vi "Parse CfgTable(with DataName).vi"(5 "Format":string, 6 "Array delimiters (|)":string="|", 7 "Cluster Configuration Typedef":variant, 8 "error in (no error)":errorcluster, 11 "CfgTable Row":string[](array[string])) -> (0 "error out":errorcluster, 1 "Elements":i32, 3 "Cluster Configuration Out":variant)   [LabVIEW 2017, in "ClusterCfgTable.lvlib"]
doc: "Parses a configuration table back into a cluster, using the data names recorded in the table to place each value. The cluster type comes from Cluster Configuration Typedef, and Elements reports how many elements were read."
uses:
  ClusterCfgTable.lvlib
  <vilib>/Utility/Data Type/Type Definitions/Data Type.ctl
  <vilib>/Utility/Data Type/Type Definitions/Refnum Type.ctl
  <vilib>/Utility/Data Type/NI_Data Type.lvlib
  _openG/_reuse_openG.lvlib
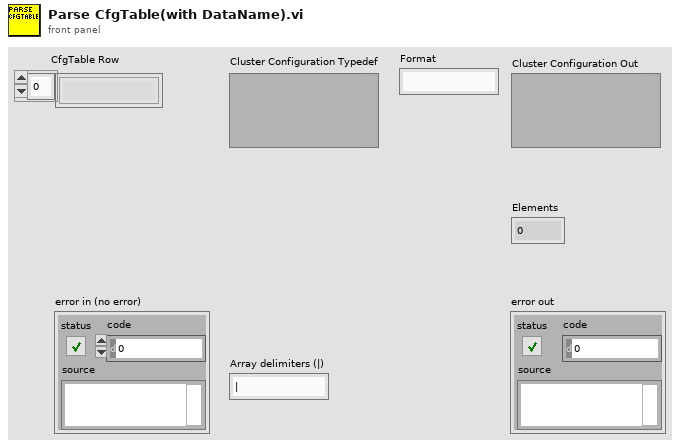
[diagram p1: front panel]
types:
  T1 = typedef "NI_Data Type.lvlib/Data Type.ctl" = enum8{"Invalid Type", "Void", "I8", "I16", "I32", "I64", "U8", "U16", "U32", "U64", "Single Float", "Double Float", "Extended Float", "Single Complex", "Double Complex", "Extended Complex", "Enum U8", "Enum U16", "Enum U32", "Enum U64", "Single Float With Unit", "Double Float With Unit", "Extended Float With Unit", "Single Complex with Unit", "Double Complex with Unit", "Extended Complex with Unit", "Boolean", "String", "Path", "Picture", "Tag", "Array", "Cluster", "Variant", "LV Variant", "Waveform", "Timestamp", "Digital Waveform", "Digital Data", "ExpressData", "Refnum", "External Data", "VI", "Poly VI", "LabVIEW Class Instance", "Fixed Point"}
  T2 = typedef "NI_Data Type.lvlib/Refnum Type.ctl" = enum16{"NotARefnum", "UnknownRefnum", "Generic", "Datalog", "ByteStream", "Device", "Occurence", "TCPNetConnection", "Auto", "Menu", "Imaq", "Hardware", "DataSocket", "Visa", "IVI", "UDPNetConnection", "Notifier", "Queue", "Irda", "EventReg", "DotNet", "UserEvent", "Callback", "UNUSED_EMPTY_POSITION", "BlueToothNetConnection", "LVObjApp", "LVObjVI", "LVObjUnknown", "GenericClass", "UserDefinedRefnumTag", "DataValue", "RT FIFO", "TDMS File"}
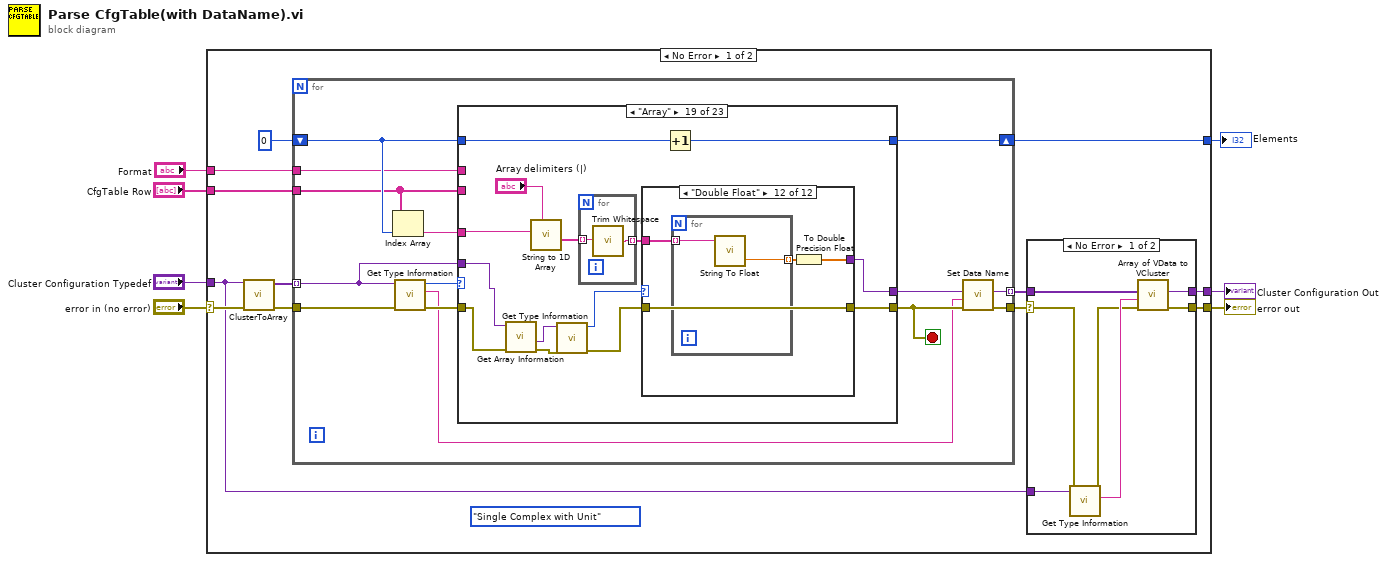
[diagram p0: block diagram]
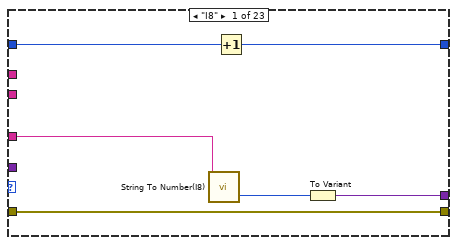
[diagram p3: hidden frame]
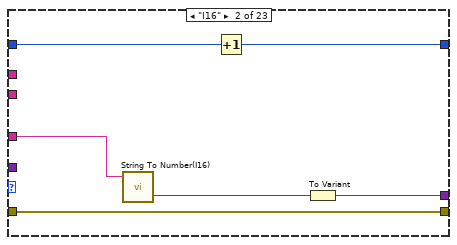
[diagram p4: hidden frame]
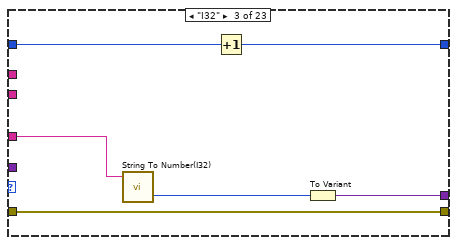
[diagram p5: hidden frame]
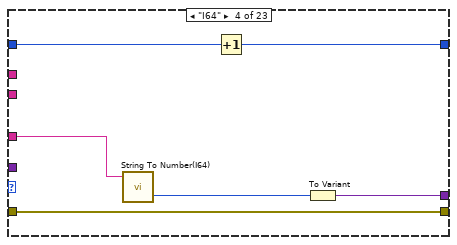
[diagram p6: hidden frame]
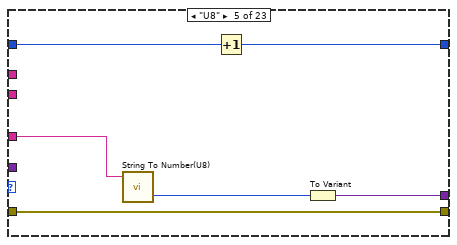
[diagram p7: hidden frame]
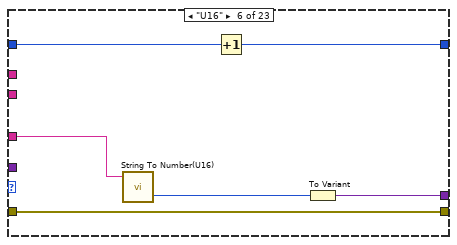
[diagram p8: hidden frame]
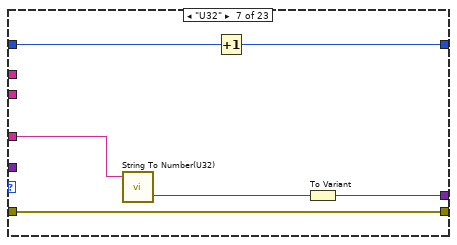
[diagram p9: hidden frame]
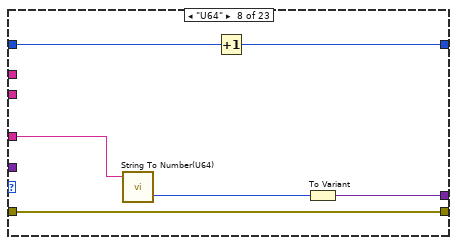
[diagram p10: hidden frame]
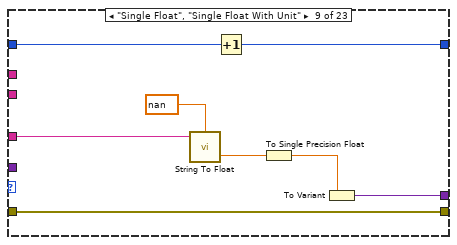
[diagram p11: hidden frame]
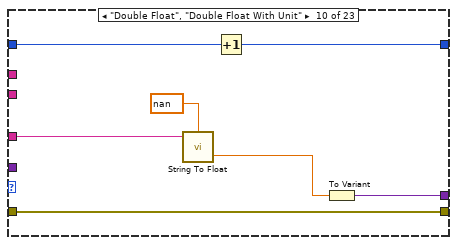
[diagram p12: hidden frame]
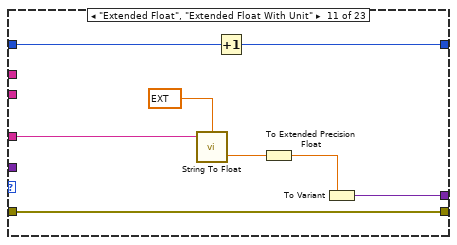
[diagram p13: hidden frame]
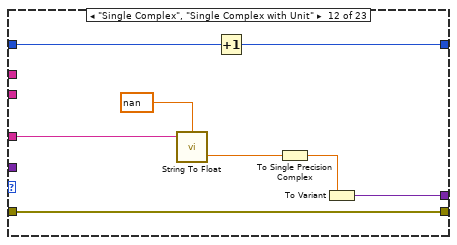
[diagram p14: hidden frame]
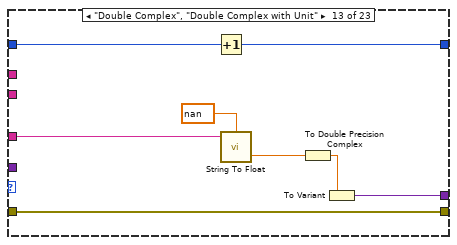
[diagram p15: hidden frame]
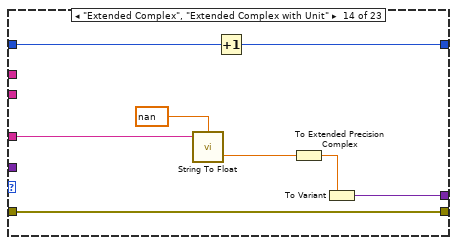
[diagram p16: hidden frame]
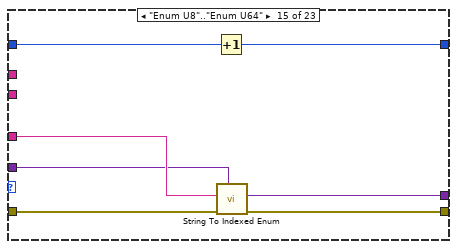
[diagram p17: hidden frame]
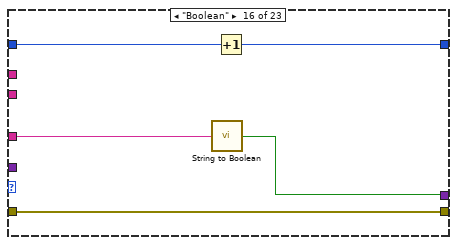
[diagram p18: hidden frame]
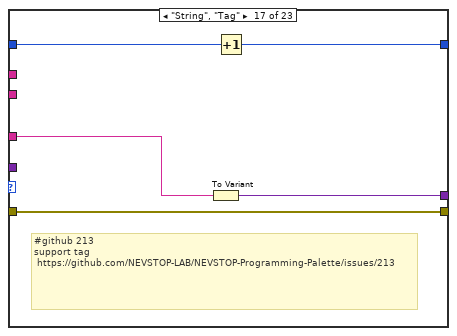
[diagram p19: hidden frame]
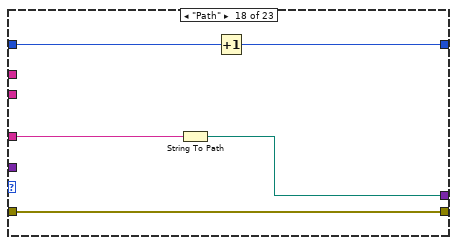
[diagram p20: hidden frame]
diagram:
  n1 = case shown="No Error" "error in (no error)" {
    selector: "error in (no error)" -> [w14 w284]
    tunnel: "CfgTable Row" -> [w19 _]
    tunnel: [w18 w283] -> w6
    tunnel: [w17 w284] -> w5
    tunnel: "Cluster Configuration Typedef" -> [w10 w283]
    tunnel: [w9 _] -> w2
    tunnel: "Format" -> [w8 _]
    frame No Error {
      (unwired) Data_Type."Single Complex with Unit" ("Type")
      n2 = call "ClusterToArray.vi"("Error in"=w14, "Cluster"=w10) -> ("Error out"=w15:errorcluster, "Array"=w12:variant[])  [unwired: 8 in]
      n3 = for {
        tunnel: w19 -> [w38]
        tunnel: w12 -> [w34] mode=indexing
        tunnel: [w37] -> w13 mode=indexing
        tunnel: w15 -> [w32]
        tunnel: [w35] -> w16
        shift-right: [w40] -> w9
        shift-left: 0 -> [w39]
        tunnel: w8 -> [w30]
        stop <- w36 stop-if-true
        n4 = Index Array(array=w38, index=w39) -> (element=w42:string)
        n5 = call <vilib>:"Get Type Information.vi"("error in (no error)"=w32, "Variant"=w34) -> ("error out"=w31:errorcluster, "Name"=w29:string, "Type"=w33:T1)  [unwired: 5 in, 2 out]
        n6 = case shown="\"Array\"" w33 {
          tunnel: w42 -> [w43 w49 w55 w61 w67 w73 w79 w85 w97 w100 w112 w120 w128 w136 w144 w149 w154 w157 w171 _ w250 w260 _]
          tunnel: [w48 w54 w60 w66 w72 w78 w84 w90 w98 w105 w113 w121 w129 w137 w143 w148 w153 w156 w168 w239 w251 w261 w277] -> w41
          tunnel: w34 -> [_ _ _ _ _ _ _ _ _ _ _ _ _ _ w142 _ _ _ w162 w240 _ w262 w277]
          tunnel: w31 -> [w46 w52 w58 w64 w70 w76 w82 w88 w96 w104 w111 w119 w127 w135 w141 w147 w152 w155 w163 w243 w245 w267 w282]
          tunnel: [w46 w52 w58 w64 w70 w76 w82 w88 w96 w104 w111 w119 w127 w135 w140 w147 w152 w155 w166 w236 w244 w266 w281] -> w36
          tunnel: w39 -> [w45 w51 w57 w63 w69 w75 w81 w87 w95 w103 w110 w118 w126 w134 w139 w146 w151 w159 w173 w238 w249 w265 w276]
          tunnel: [w44 w50 w56 w62 w68 w74 w80 w86 w94 w102 w109 w117 w125 w133 w138 w145 w150 w158 w172 w237 w248 w265 w276] -> w40
          tunnel: w38 -> [_ _ _ _ _ _ _ _ _ _ _ _ _ _ _ _ _ _ _ w242 _ _ _]
          tunnel: w30 -> [_ _ _ _ _ _ _ _ _ _ _ _ _ _ _ _ _ _ _ _ w246 _ _]
          frame "I8" {
            n7 = call "String To Number(I8).vi"("String"=w43) -> ("Numeric(I8)"=w47:i8)  [unwired: 4 in]
            n8 = Increment(x=w45) -> (x+1=w44:i32)
            n9 = To Variant(anything=w47) -> (Variant=w48:variant)
          }
          frame "I16" {
            n10 = call "String To Number(I16).vi"("String"=w49) -> ("Numeric(I16)"=w53:i16)  [unwired: 4 in]
            n11 = Increment(x=w51) -> (x+1=w50:i32)
            n12 = To Variant(anything=w53) -> (Variant=w54:variant)
          }
          frame "I32" {
            n13 = call "String To Number(I32).vi"("String"=w55) -> ("Numeric(I32)"=w59:i32)  [unwired: 4 in]
            n14 = Increment(x=w57) -> (x+1=w56:i32)
            n15 = To Variant(anything=w59) -> (Variant=w60:variant)
          }
          frame "I64" {
            n16 = call "String To Number(I64).vi"("String"=w61) -> ("Numeric(I64)"=w65:i64)  [unwired: 4 in]
            n17 = Increment(x=w63) -> (x+1=w62:i32)
            n18 = To Variant(anything=w65) -> (Variant=w66:variant)
          }
          frame "U8" {
            n19 = call "String To Number(U8).vi"("String"=w67) -> ("Numeric(U8)"=w71:u8)  [unwired: 4 in]
            n20 = Increment(x=w69) -> (x+1=w68:i32)
            n21 = To Variant(anything=w71) -> (Variant=w72:variant)
          }
          frame "U16" {
            n22 = call "String To Number(U16).vi"("String"=w73) -> ("Numeric(U16)"=w77:u16)  [unwired: 4 in]
            n23 = Increment(x=w75) -> (x+1=w74:i32)
            n24 = To Variant(anything=w77) -> (Variant=w78:variant)
          }
          frame "U32" {
            n25 = call "String To Number(U32).vi"("String"=w79) -> ("Numeric(U32)"=w83:u32)  [unwired: 4 in]
            n26 = Increment(x=w81) -> (x+1=w80:i32)
            n27 = To Variant(anything=w83) -> (Variant=w84:variant)
          }
          frame "U64" {
            n28 = call "String To Number(U64).vi"("String"=w85) -> ("Numeric(U64)"=w89:u64)  [unwired: 4 in]
            n29 = Increment(x=w87) -> (x+1=w86:i32)
            n30 = To Variant(anything=w89) -> (Variant=w90:variant)
          }
          frame "Single Float", "Single Float With Unit" {
            n31 = call "String To Float.vi"("Default(0)"=nan ("number"), "String"=w97) -> ("Float"=w93:dbl)  [unwired: 3 in]
            n32 = Increment(x=w95) -> (x+1=w94:i32)
            n33 = To Single Precision Float(number=w93) -> (single precision float=w92:sgl)
            n34 = To Variant(anything=w92) -> (Variant=w98:variant)
          }
          frame "Double Float", "Double Float With Unit" {
            n35 = call "String To Float.vi"("Default(0)"=nan ("number"), "String"=w100) -> ("Float"=w99:dbl)  [unwired: 3 in]
            n36 = Increment(x=w103) -> (x+1=w102:i32)
            n37 = To Variant(anything=w99) -> (Variant=w105:variant)
          }
          frame "Extended Float", "Extended Float With Unit" {
            n38 = call "String To Float.vi"("Default(0)"=ext nan ("number"), "String"=w112) -> ("Float"=w108:dbl)  [unwired: 3 in]
            n39 = Increment(x=w110) -> (x+1=w109:i32)
            n40 = To Extended Precision Float(1:w108) -> (0:w107:ext)
            n41 = To Variant(anything=w107) -> (Variant=w113:variant)
          }
          frame "Single Complex", "Single Complex with Unit" {
            n42 = call "String To Float.vi"("Default(0)"=nan ("number"), "String"=w120) -> ("Float"=w116:dbl)  [unwired: 3 in]
            n43 = Increment(x=w118) -> (x+1=w117:i32)
            n44 = To Single Precision Complex(1:w116) -> (0:w115:csg)
            n45 = To Variant(anything=w115) -> (Variant=w121:variant)
          }
          frame "Double Complex", "Double Complex with Unit" {
            n46 = Increment(x=w126) -> (x+1=w125:i32)
            n47 = call "String To Float.vi"("Default(0)"=nan ("number"), "String"=w128) -> ("Float"=w124:dbl)  [unwired: 3 in]
            n48 = To Double Precision Complex(1:w124) -> (0:w123:cdb)
            n49 = To Variant(anything=w123) -> (Variant=w129:variant)
          }
          frame "Extended Complex", "Extended Complex with Unit" {
            n50 = call "String To Float.vi"("Default(0)"=nan ("number"), "String"=w136) -> ("Float"=w132:dbl)  [unwired: 3 in]
            n51 = Increment(x=w134) -> (x+1=w133:i32)
            n52 = To Extended Precision Complex(1:w132) -> (0:w131:cxt)
            n53 = To Variant(anything=w131) -> (Variant=w137:variant)
          }
          frame "Enum U8".."Enum U64" {
            n54 = Increment(x=w139) -> (x+1=w138:i32)
            n55 = call "String To Indexed Enum.vi"("Variant"=w142, "error in (no error)"=w141, "String"=w144) -> ("error out"=w140:errorcluster, "Enum"=w143:variant)  [unwired: 7 in]
          }
          frame "Boolean" {
            n56 = call "String to Boolean.vi"("String"=w149) -> ("Boolean"=w148:bool)  [unwired: 3 in]
            n57 = Increment(x=w146) -> (x+1=w145:i32)
          }
          frame "String", "Tag" {
            # "#github 213\nsupport tag\n https://github.com/NEVSTOP-LAB/NEVSTOP-Programming-Palette/issues/213"
            n58 = To Variant(anything=w154) -> (Variant=w153:variant)
            n59 = Increment(x=w151) -> (x+1=w150:i32)
          }
          frame "Path" {
            n60 = String To Path(string=w157) -> (path=w156:path)
            n61 = Increment(x=w159) -> (x+1=w158:i32)
          }
          frame "Array" {
            n62 = call <vilib>:"Get Array Information.vi"("error in (no error)"=w163, "Variant"=w162) -> ("error out"=w165:errorcluster, "Array Element Data Type"=w164:variant)  [unwired: 6 in, 2 out]
            n63 = call "String to 1D Array.vi"("delimiter (Tab)"="Array delimiters (|)", "string"=w171) -> ("Array of Strings"=w169:string[])  [unwired: 9 in]
            n64 = call <vilib>:"Get Type Information.vi"("error in (no error)"=w165, "Variant"=w164) -> ("error out"=w161:errorcluster, "Type"=w160:T1)  [unwired: 5 in, 3 out]
            n65 = for {
              tunnel: w169 -> [w175] mode=indexing
              tunnel: [w174] -> w167 mode=indexing
              n66 = call <vilib>:"Trim Whitespace.vi"("string"=w175) -> ("trimmed string"=w174:string)  [unwired: 1 in]
            }
            n67 = case shown="\"Double Float\"" w160 {
              tunnel: [w179 w180 w183 w188 w193 w198 w203 w208 w213 w218 w223 w229] -> w168
              tunnel: w167 -> [w179 w182 w185 w190 w195 w200 w205 w210 w215 w220 w226 w232]
              tunnel: [w176 w181 w184 w189 w194 w199 w204 w209 w214 w219 w225 w231] -> w166
              tunnel: w161 -> [_ w181 w184 w189 w194 w199 w204 w209 w214 w219 w225 w231]
              frame "Invalid Type", Default {
                n68 = call "Error From Error Code.vi"("error message (\"\")"="Input Config Contains unsupported datatype" ("String to Prepend to source (\"\")"), "error code (0)"=1 ("code")) -> ("error out"=w176:errorcluster)  [unwired: 7 in]
              }
              frame "String" {
                n69 = To Variant(anything=w182) -> (Variant=w180:variant)
              }
              frame "U8" {
                n70 = for {
                  tunnel: w185 -> [w187] mode=indexing
                  tunnel: [w186] -> w183 mode=indexing
                  n71 = call "String To Number(U8).vi"("String"=w187) -> ("Numeric(U8)"=w186:u8)  [unwired: 4 in]
                }
              }
              frame "U16" {
                n72 = for {
                  tunnel: w190 -> [w192] mode=indexing
                  tunnel: [w191] -> w188 mode=indexing
                  n73 = call "String To Number(U16).vi"("String"=w192) -> ("Numeric(U16)"=w191:u16)  [unwired: 4 in]
                }
              }
              frame "U32" {
                n74 = for {
                  tunnel: w195 -> [w197] mode=indexing
                  tunnel: [w196] -> w193 mode=indexing
                  n75 = call "String To Number(U32).vi"("String"=w197) -> ("Numeric(U32)"=w196:u32)  [unwired: 4 in]
                }
              }
              frame "U64" {
                n76 = for {
                  tunnel: w200 -> [w202] mode=indexing
                  tunnel: [w201] -> w198 mode=indexing
                  n77 = call "String To Number(U64).vi"("String"=w202) -> ("Numeric(U64)"=w201:u64)  [unwired: 4 in]
                }
              }
              frame "I8" {
                n78 = for {
                  tunnel: w205 -> [w207] mode=indexing
                  tunnel: [w206] -> w203 mode=indexing
                  n79 = call "String To Number(I8).vi"("String"=w207) -> ("Numeric(I8)"=w206:i8)  [unwired: 4 in]
                }
              }
              frame "I16" {
                n80 = for {
                  tunnel: w210 -> [w212] mode=indexing
                  tunnel: [w211] -> w208 mode=indexing
                  n81 = call "String To Number(I16).vi"("String"=w212) -> ("Numeric(I16)"=w211:i16)  [unwired: 4 in]
                }
              }
              frame "I32" {
                n82 = for {
                  tunnel: w215 -> [w217] mode=indexing
                  tunnel: [w216] -> w213 mode=indexing
                  n83 = call "String To Number(I32).vi"("String"=w217) -> ("Numeric(I32)"=w216:i32)  [unwired: 4 in]
                }
              }
              frame "I64" {
                n84 = for {
                  tunnel: w220 -> [w222] mode=indexing
                  tunnel: [w221] -> w218 mode=indexing
                  n85 = call "String To Number(I64).vi"("String"=w222) -> ("Numeric(I64)"=w221:i64)  [unwired: 4 in]
                }
              }
              frame "Single Float" {
                n86 = for {
                  tunnel: w226 -> [w228] mode=indexing
                  tunnel: [w227] -> w224 mode=indexing
                  n87 = call "String To Float.vi"("String"=w228) -> ("Float"=w227:dbl)  [unwired: 4 in]
                }
                n88 = To Single Precision Float(number=w224) -> (single precision float=w223:sgl[])
              }
              frame "Double Float" {
                n89 = for {
                  tunnel: w232 -> [w234] mode=indexing
                  tunnel: [w233] -> w230 mode=indexing
                  n90 = call "String To Float.vi"("String"=w234) -> ("Float"=w233:dbl)  [unwired: 4 in]
                }
                n91 = To Double Precision Float(number=w230) -> (double precision float=w229:dbl[])
              }
            }
            n92 = Increment(x=w173) -> (x+1=w172:i32)
          }
          frame "Cluster" {
            n93 = Array Subset(array=w242, index=w238) -> (w241:string[])  [unwired: 1 in]
            n94 = call "Parse CfgTable(with DataName).vi"("Cluster Configuration Typedef"=w240, "error in (no error)"=w243, "CfgTable Row"=w241) -> ("error out"=w236:errorcluster, "Elements"=w235:i32, "Cluster Configuration Out"=w239:variant)  [unwired: 6 in]
            n95 = Add(x=w238, y=w235) -> (x+y=w237:i32)
          }
          frame "Timestamp" {
            n96 = case shown="Default" w250 {
              selector: w250 -> [_ w259]
              tunnel: [timestamp(0 s since 1904-01-01) ("Time Stamp") w257] -> w247
              tunnel: w246 -> [_ w258]
              tunnel: w245 -> [w252 w255]
              tunnel: [w252 w254] -> w244
              frame "" {
              }
              frame Default {
                n97 = Scan From String(format string=w258, input string=w259, error in=w255, default 1=timestamp(0 s since 1904-01-01) ("Time Stamp")) -> (error out=w254:errorcluster, output 1=w257:timestamp)  [unwired: 1 in, 2 out]
              }
            }
            n98 = Increment(x=w249) -> (x+1=w248:i32)
            n99 = To Variant(anything=w247) -> (Variant=w251:variant)
          }
          frame "Refnum" {
            n100 = call <vilib>:"Get Refnum Information.vi"("error in (no error)"=w267, "Variant"=w262) -> ("error out"=w264:errorcluster, "Reference Type"=w263:T2)  [unwired: 6 in, 2 out]
            n101 = case shown="Default" w263 {
              tunnel: [w269 w275] -> w266
              tunnel: w264 -> [w269 w271]
              tunnel: w262 -> [_ w270]
              tunnel: [w268 w270] -> w261
              tunnel: w260 -> [w268 _]
              frame "UserDefinedRefnumTag" {
                (unwired) Refnum_Type."NotARefnum" ("Reference Type")
              }
              frame Default {
                n102 = call "Error From Error Code.vi"("error message (\"\")"="Input Config Contains unsupported datatype" ("String to Prepend to source (\"\")"), "error code (0)"=1 ("code")) -> ("error out"=w274:errorcluster)  [unwired: 7 in]
                n103 = Merge Errors(w271, w274) -> (w275:errorcluster)
              }
            }
          }
          frame Default {
            n104 = call "Error From Error Code.vi"("error message (\"\")"="Input Config Contains unsupported datatype" ("String to Prepend to source (\"\")"), "error code (0)"=1 ("code")) -> ("error out"=w280:errorcluster)  [unwired: 7 in]
            n105 = Merge Errors(w282, w280) -> (w281:errorcluster)
          }
        }
        n106 = call "Set Data Name.vi"("error in (no error)"=w36, "Data Name"=w29, "Data"=w41) -> ("error out"=w35:errorcluster, "Renamed Data"=w37:variant)  [unwired: 7 in]
      }
      n107 = case shown="No Error" w16 {
        selector: w16 -> [w21 w27]
        tunnel: [w26 w28] -> w18
        tunnel: [w25 w27] -> w17
        tunnel: w13 -> [w24 _]
        tunnel: w10 -> [w22 w28]
        frame No Error {
          n108 = call <vilib>:"Get Type Information.vi"("error in (no error)"=w21, "Variant"=w22) -> ("error out"=w20:errorcluster, "Name"=w23:string)  [unwired: 5 in, 3 out]
          n109 = call "Array of VData to VCluster.vi"("error in (no error)"=w20, "Cluster Name"=w23, "Array"=w24) -> ("error out"=w25:errorcluster, "VCluster"=w26:variant)  [unwired: 7 in]
        }
        frame Error {
        }
      }
    }
    frame Error {
    }
  }
  "Cluster Configuration Out" <- w6
  "error out" <- w5
  "Elements" <- w2
